vi "Read Info.vi"(8 "error in (no error)":errorcluster, 11 "Git Updater Module in":refnum<class "Git Updater Module.lvclass">) -> (0 "error out":errorcluster, 2 "Git Info":T1, 3 "Git Updater Module out":refnum<class "Git Updater Module.lvclass">)   [LabVIEW 2020, in "VolatusGUI.lvlib" / "Git Updater Module.lvclass"]
uses:
  Git Updater Module.lvclass
  Git Info.ctl
  <vilib>/Hampel Software Engineering/Git API/Git API/Controls/GIT-Repository States.ctl
  <vilib>/Hampel Software Engineering/Git API/Git API/GIT-api.lvclass/GIT-api.ctl
  Git Updater Module.lvclass/Git Updater Module.ctl
  <vilib>/Hampel Software Engineering/Git API/Git API/GIT-api.lvclass
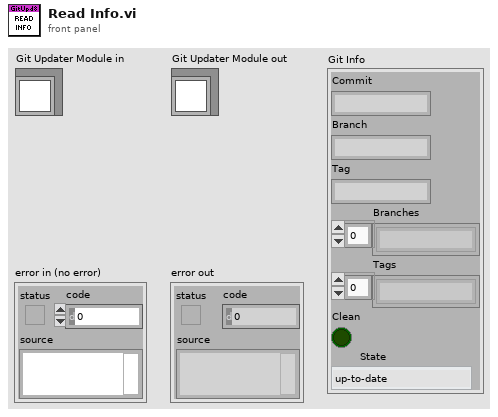
[diagram p1: front panel]
types:
  T1 = typedef "VolatusGUI.lvlib/Git Updater Module.lvclass/Git Info.ctl" = cluster{"Commit":string, "Branch":string, "Tag":string, "Branches":string[], "Tags":string[], "Clean":bool, "State":T2}
  T2 = typedef "GIT-API-for-LabVIEW.lvlib/GIT-api.lvclass/GIT-Repository States.ctl" = enum16{"up-to-date", "behind", "ahead", "diverged", "unpublished", "detached", "unknown"}
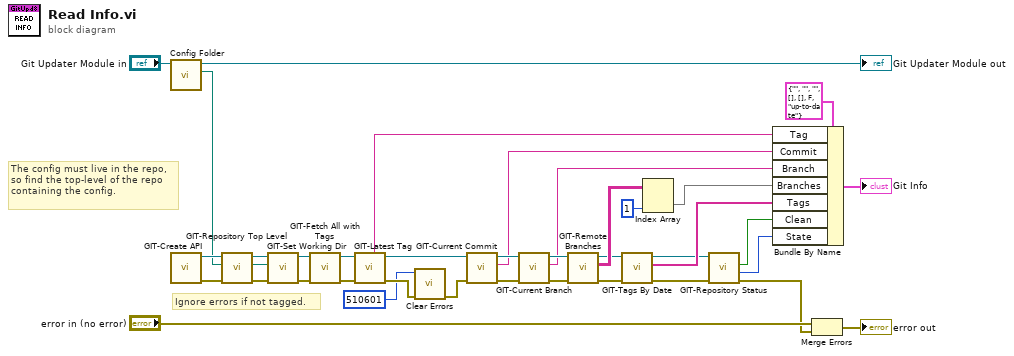
[diagram p0: block diagram]
diagram:
  # "The config must live in the repo, so find the top-level of the repo containing the config."
  # "Ignore errors if not tagged."
  n1 = call "Config Folder.vi"("Git Updater Module in"="Git Updater Module in") -> ("Config Folder"=w1:path, "Git Updater Module out"=→"Git Updater Module out":refnum<class "Git Updater Module.lvclass">)  [unwired: 8 in, 1 out]
  n2 = call <vilib>:"GIT-Create API.vi"() -> ("error out"=w37:errorcluster, "git-api out"=w38:refnum<class "GIT-api.lvclass">)  [unwired: 10 in]
  n3 = call <vilib>:"GIT-Repository Top Level.vi"("error in"=w37, "Current Path"=w1, "git-api in"=w38) -> ("error out"=w34:errorcluster, "Repo Top Level Path"=w35:path, "git-api out"=w36:refnum<class "GIT-api.lvclass">)  [unwired: 6 in]
  n4 = call <vilib>:"GIT-Set Working Dir.vi"("error in"=w34, "Working Directory"=w35, "git-api in"=w36) -> ("error out"=w33:errorcluster, "git-api out"=w19:refnum<class "GIT-api.lvclass">)  [unwired: 7 in]
  n5 = call <vilib>:"GIT-Fetch All with Tags.vi"("error in"=w33, "Git-API in"=w19) -> ("error out"=w20:errorcluster, "Git-API out"=w18:refnum<class "GIT-api.lvclass">)  [unwired: 8 in]
  n6 = call <vilib>:"GIT-Latest Tag.vi"("error in"=w20, "git-api in"=w18) -> ("error out"=w29:errorcluster, "git-api out"=w32:refnum<class "GIT-api.lvclass">, "Latest Tag"=w14:string)  [unwired: 6 in, 1 out]
  n7 = call <vilib>:"Clear Errors.vi"("error in (no error)"=w29, "specific error code to clear (0: all)"=510601) -> ("error out"=w28:errorcluster)  [unwired: 4 in, 1 out]
  n8 = call <vilib>:"GIT-Current Commit.vi"("error in"=w28, "git-api in"=w32) -> ("error out"=w30:errorcluster, "current commit"=w13:string, "git-api out"=w31:refnum<class "GIT-api.lvclass">)  [unwired: 7 in]
  n9 = call <vilib>:"GIT-Current Branch.vi"("error in"=w30, "git-api in"=w31) -> ("error out"=w26:errorcluster, "current branch"=w12:string, "git-api out"=w25:refnum<class "GIT-api.lvclass">)  [unwired: 6 in, 1 out]
  n10 = call <vilib>:"GIT-Remote Branches.vi"("error in"=w26, "git-api in"=w25) -> ("error out"=w22:errorcluster, "branches"=w24:string[][], "git-api out"=w21:refnum<class "GIT-api.lvclass">)  [unwired: 7 in]
  n11 = call <vilib>:"GIT-Tags By Date.vi"("error in"=w22, "Git-API in"=w21) -> ("error out"=w6:errorcluster, "tags"=w10:string[], "Git-API out"=w5:refnum<class "GIT-api.lvclass">)  [unwired: 7 in]
  n12 = Index Array(array=w24, index (col)=1 ("disabled index (col)")) -> (element=w11:string[])  [unwired: 1 in]
  n13 = call <vilib>:"GIT-Repository Status.vi"("error in"=w6, "git-api in"=w5) -> ("error out"=w2:errorcluster, "State"=w3:T2, "Clean?"=w4:bool)  [unwired: 6 in, 1 out]
  n14 = Bundle By Name(cluster=T1 {"Commit"="", "Branch"="", "Tag"="", "Branches"=[], "Tags"=[], "Clean"=FALSE, "State"=enum."up-to-date"} ("Git Info"), "Tag"=w14, "Commit"=w13, "Branch"=w12, "Branches"=w11, "Tags"=w10, "Clean"=w4, "State"=w3) -> (→"Git Info":T1)
  n15 = Merge Errors("error in (no error)", w2) -> (→"error out":errorcluster)
